vi "test_Get Bitfile Scalars.vi"(8 "error in (no error)":errorcluster, 11 "TestCase in":refnum<class "FPGA Addon Scripting API Unit Tests.lvclass">) -> (0 "error out":errorcluster, 3 "TestCase out":refnum<class "FPGA Addon Scripting API Unit Tests.lvclass">)   [LabVIEW 2020, in "FPGA Addon Scripting API Unit Tests.lvclass"]
uses:
  FPGA Addon Scripting API Unit Tests.lvclass
  APIs/Scripting API/TypeDefs/Output Scalar Data.ctl
  Addon/Addon Shared/Types/FPGA Addon Data Type.ctl
  <vilib>/addons/_JKI Toolkits/VI Tester/TestCase.llb/TestCase.lvclass
  FPGA Addon Test Class/FPGA Addon Test Class.lvclass
  APIs/Scripting API/Scripting API.lvlib
  Addon/Addon Shared/FPGA Addon Shared.lvlib
  C:/Program Files (x86)/National Instruments/LabVIEW 2020/vi.lib/addons/_JKI Toolkits/VI Tester/TestCase.llb/TestCase.lvclass
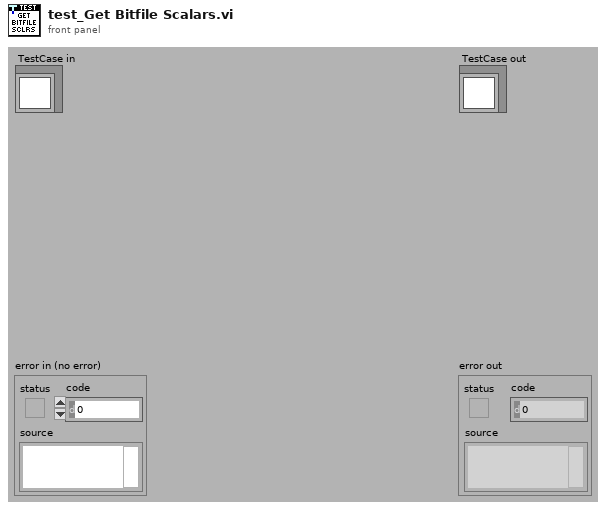
[diagram p1: front panel]
types:
  T1 = typedef "Scripting API.lvlib/Output Scalar Data.ctl" = cluster{"Bitfile Name":string, "SysDef Channel Name":string, "Imported":bool, "Data Type":T2}
  T2 = typedef "FPGA Addon Shared.lvlib/FPGA Addon Data Type.ctl" = enum8{"<Null>", "I8", "I16", "I32", "I64", "U8", "U16", "U32", "U64", "SGL", "Boolean", "Analog PWM In Settings", "Analog PWM In", "Digital PWM In Settings", "Digital PWM In", "Digital PWM Out", "Sine Out", "FXP", "FXP+/-24.5", "FXP+/-16.5", "FXP+/-32.8", "FXP+/-64.32", "FXP+/-16.7", "FXP+/-20.5", "FXP+/-27.5", "FXP+/-32.16", "FXP+16.3", "FXP+18.3", "Digital Static In", "Digital Static Out", "Digital Static In Settings", "Digital WSS Out", "Quad Encoder Settings", "Quad Encoder In", "Group"}
  T3 = typedef "Custom Device API.lvlib/Custom Device Item Ref.ctl" = u64
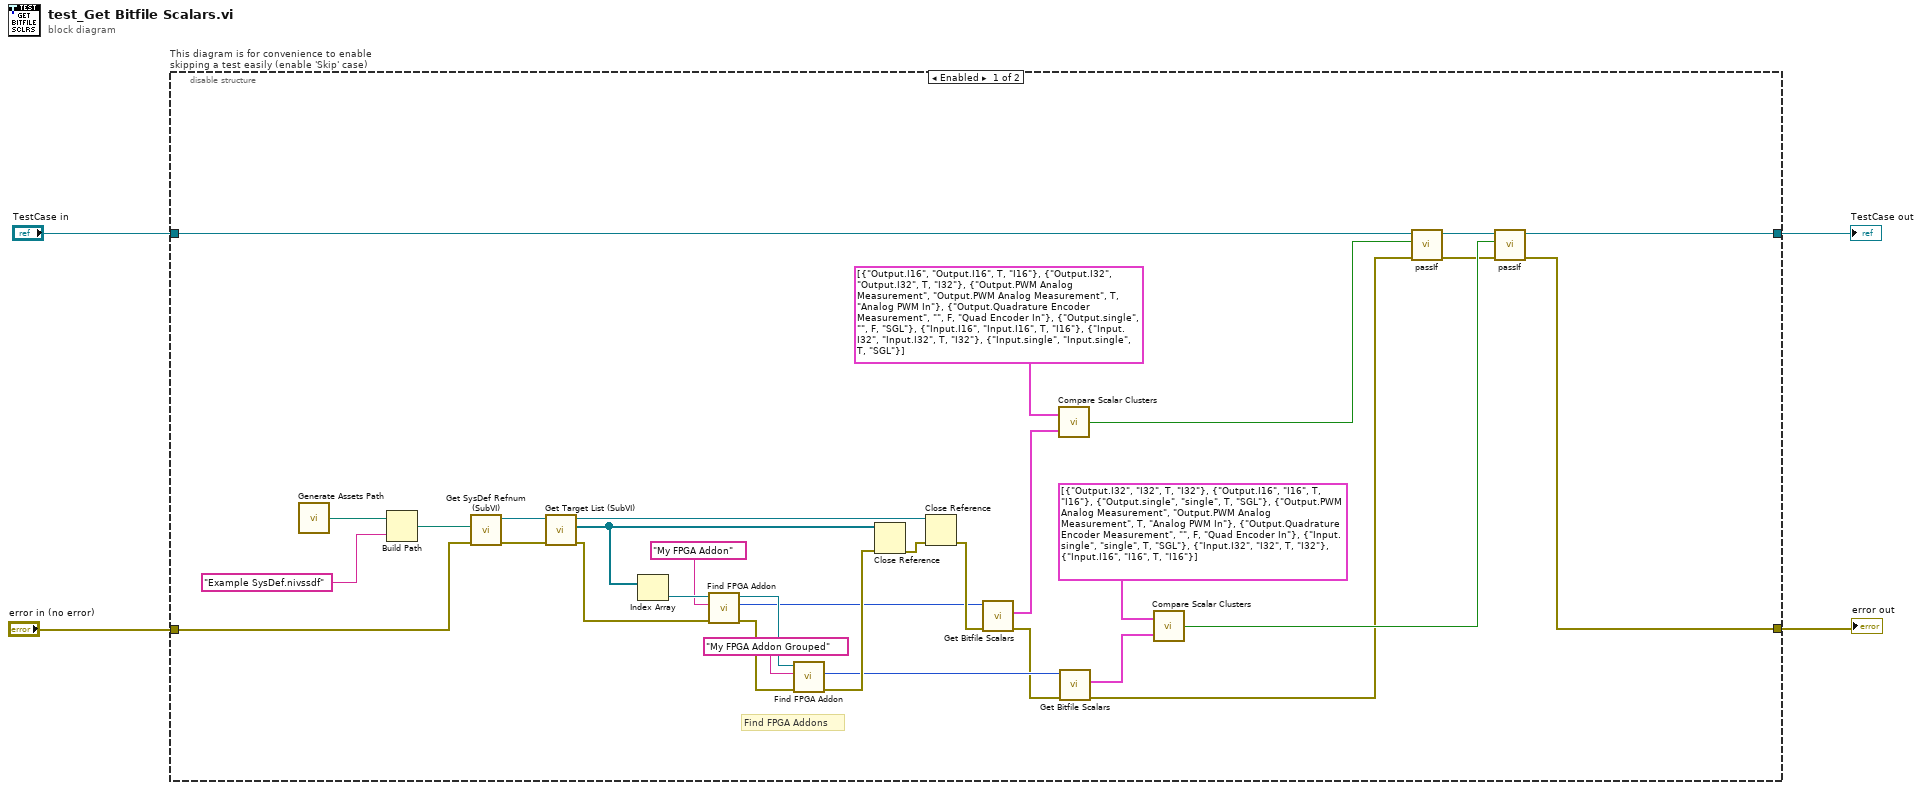
[diagram p0: block diagram]
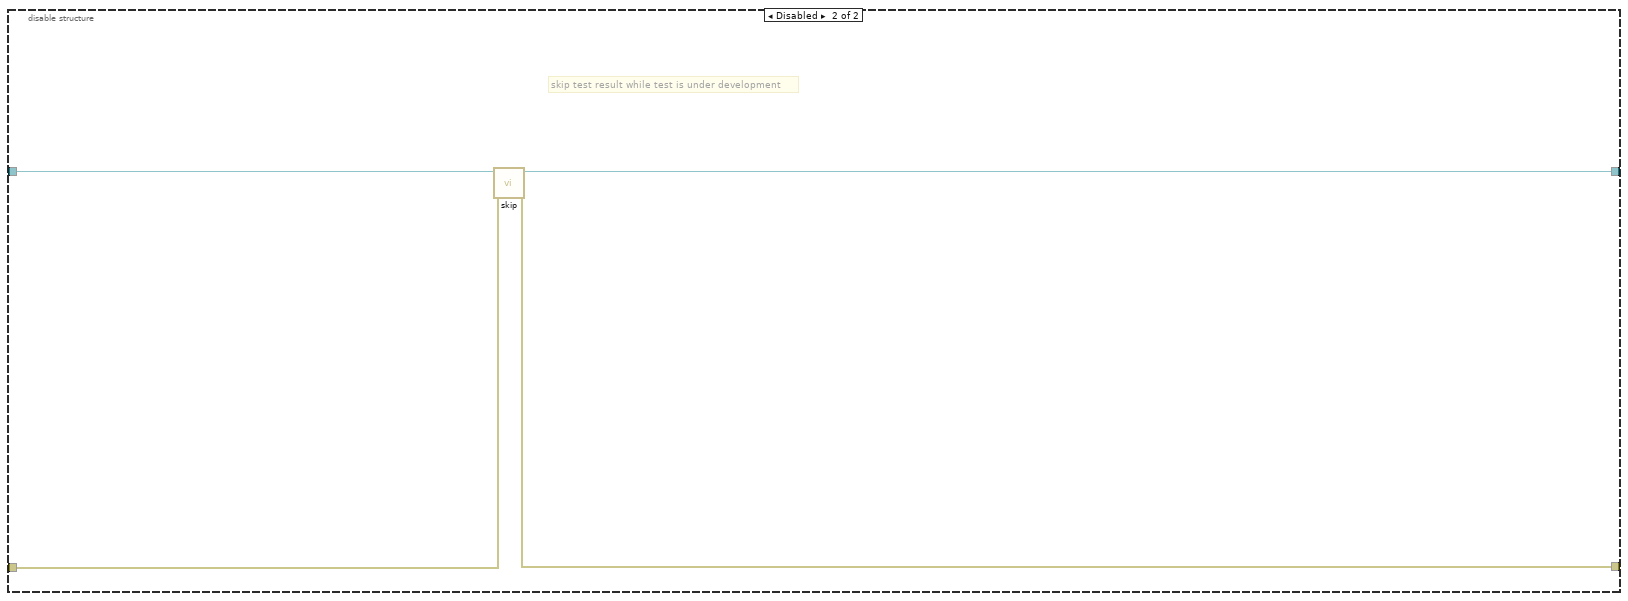
[diagram p2: hidden frame]
diagram:
  n1 = disable-structure "This diagram is for convenience to enable skipping a test easily (enable 'Skip' case)" shown="Enabled" {
    disable-tunnel: "TestCase in" -> [w12 w40]
    disable-tunnel: [w5 w38] -> w1
    disable-tunnel: [w6 w39] -> w3
    disable-tunnel: "error in (no error)" -> [w32 w37]
    frame Enabled {
      # "Find FPGA Addons"
      n2 = call "Generate Assets Path.vi"() -> ("Assets path"=w36:path)
      n3 = Build Path(base path=w36, name or relative path="Example SysDef.nivssdf") -> (appended path=w34:path)
      n4 = call "Get SysDef Refnum (SubVI).vi"("error in (no error)"=w32, "System Definition path"=w34) -> ("error out"=w31:errorcluster, "SysDef Refnum out"=w33:refnum<k24>)  [unwired: 8 in]
      n5 = call "Get Target List (SubVI).vi"("error in (no error)"=w31, "SysDef Refnum in"=w33) -> ("error out"=w26:errorcluster, "Target List Refnums"=w30:refnum<k24>[], "SysDef Refnum out"=w29:refnum<k24>)  [unwired: 7 in]
      n6 = Index Array(array=w30) -> (element=w27:refnum<k24>)  [unwired: 1 in]
      n7 = call "Find FPGA Addon.vi"("error in"=w26, "FPGA addon name"="My FPGA Addon", "target in"=w27) -> ("error out"=w21:errorcluster, "FPGA addon refnum out"=w17:T3, "target out"=w20:refnum<k24>)  [unwired: 5 in, 1 out]
      n8 = call "Find FPGA Addon.vi"("error in"=w21, "FPGA addon name"="My FPGA Addon Grouped", "target in"=w20) -> ("error out"=w18:errorcluster, "FPGA addon refnum out"=w16:T3)  [unwired: 5 in, 2 out]
      n9 = Close Reference(reference=w30, error in (no error)=w18) -> (error out=w28:errorcluster)
      n10 = Close Reference(reference=w29, error in (no error)=w28) -> (error out=w24:errorcluster)
      n11 = call "Get Bitfile Scalars.vi"("error in"=w24, "FPGA addon refnum in"=w17) -> ("error out"=w15:errorcluster, "bitfile scalars out"=w23:T1[])  [unwired: 7 in, 1 out]
      n12 = call "Compare Scalar Clusters.vi"("Target bitfile scalars in"=w23, "Reference bitfile scalars in"=T1[] [{"Bitfile Name"="Output.I16", "SysDef Channel Name"="Output.I16", "Imported"=TRUE, "Data Type"=enum."I16"}, {"Bitfile Name"="Output.I32", "SysDef Channel Name"="Output.I32", "Imported"=TRUE, "Data Type"=enum."I32"}, {"Bitfile Name"="Output.PWM Analog Measurement", "SysDef Channel Name"="Output.PWM Analog Measurement", "Imported"=TRUE, "Data Type"=enum."Analog PWM In"}, {"Bitfile Name"="Output.Quadrature Encoder Measurement", "SysDef Channel Name"="", "Imported"=FALSE, "Data Type"=enum."Quad Encoder In"}, {"Bitfile Name"="Output.single", "SysDef Channel Name"="", "Imported"=FALSE, "Data Type"=enum."SGL"}, {"Bitfile Name"="Input.I16", "SysDef Channel Name"="Input.I16", "Imported"=TRUE, "Data Type"=enum."I16"}, {"Bitfile Name"="Input.I32", "SysDef Channel Name"="Input.I32", "Imported"=TRUE, "Data Type"=enum."I32"}, {"Bitfile Name"="Input.single", "SysDef Channel Name"="Input.single", "Imported"=TRUE, "Data Type"=enum."SGL"}] ("bitfile scalars out")) -> ("Equal ?"=w11:bool)
      n13 = call "Get Bitfile Scalars.vi"("error in"=w15, "FPGA addon refnum in"=w16) -> ("error out"=w8:errorcluster, "bitfile scalars out"=w14:T1[])  [unwired: 7 in, 1 out]
      n14 = call "Compare Scalar Clusters.vi"("Target bitfile scalars in"=w14, "Reference bitfile scalars in"=T1[] [{"Bitfile Name"="Output.I32", "SysDef Channel Name"="I32", "Imported"=TRUE, "Data Type"=enum."I32"}, {"Bitfile Name"="Output.I16", "SysDef Channel Name"="I16", "Imported"=TRUE, "Data Type"=enum."I16"}, {"Bitfile Name"="Output.single", "SysDef Channel Name"="single", "Imported"=TRUE, "Data Type"=enum."SGL"}, {"Bitfile Name"="Output.PWM Analog Measurement", "SysDef Channel Name"="Output.PWM Analog Measurement", "Imported"=TRUE, "Data Type"=enum."Analog PWM In"}, {"Bitfile Name"="Output.Quadrature Encoder Measurement", "SysDef Channel Name"="", "Imported"=FALSE, "Data Type"=enum."Quad Encoder In"}, {"Bitfile Name"="Input.single", "SysDef Channel Name"="single", "Imported"=TRUE, "Data Type"=enum."SGL"}, {"Bitfile Name"="Input.I32", "SysDef Channel Name"="I32", "Imported"=TRUE, "Data Type"=enum."I32"}, {"Bitfile Name"="Input.I16", "SysDef Channel Name"="I16", "Imported"=TRUE, "Data Type"=enum."I16"}] ("bitfile scalars out")) -> ("Equal ?"=w9:bool)
      n15 = call-dynamic "passIf.vi"("error in (no error)"=w8, "pass"=w11, "TestCase in"=w12) -> ("error out"=w7:errorcluster, "TestCase out"=w10:refnum<class "FPGA Addon Scripting API Unit Tests.lvclass">)  [unwired: 7 in]
      n16 = call-dynamic "passIf.vi"("error in (no error)"=w7, "pass"=w9, "TestCase in"=w10) -> ("error out"=w6:errorcluster, "TestCase out"=w5:refnum<class "FPGA Addon Scripting API Unit Tests.lvclass">)  [unwired: 7 in]
    }
    frame Disabled {
      # "skip test result while test is under development"
      n17 = call <vilib>:"skip.vi"("error in (no error)"=w37, "TestCase in"=w40) -> ("error out"=w39:errorcluster, "TestCase out"=w38:refnum<class "FPGA Addon Scripting API Unit Tests.lvclass">)  [unwired: 8 in]
    }
  }
  "error out" <- w3
  "TestCase out" <- w1
